vi "Periodic Tasks.vi"(8 "error in":errorcluster) -> ()   [LabVIEW 2019]
doc: "This VI runs in parallel to other tasks. It can contain as many user-defined periodic loops as you need. These can carry out PID or other sorts of timed response."
uses:
  <vilib>/Rock Robotics/WPI/DriverStation/WPI_DriverStationRobotMode2.ctl
  Robot Global Data.vi
  <vilib>/Rock Robotics/WPI/Utilities/WPI_GetSetVariantRefNum.vi
  <vilib>/Rock Robotics/Network Tables/NT Write Boolean.vi
  <vilib>/Rock Robotics/Network Tables/NT Write Number.vi
  <vilib>/Rock Robotics/Network Tables/NT Read Number.vi
  <vilib>/Rock Robotics/WPI/RobotDrive/WPI_RobotDriveArcadeDrive_Standard(NoSaturation).vi
  <vilib>/Rock Robotics/Network Tables/NT Read Boolean.vi
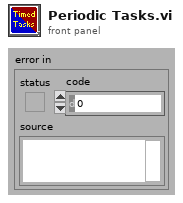
[diagram p1: front panel]
types:
  T1 = typedef "WPI_JoystickDevRef.ctl" = cluster{"Device":T2}
  T2 = typedef "WPI_JoystickDeviceEnum.ctl" = enum16{"USB 0", "USB 1", "USB 2", "USB 3", "USB 4", "USB 5"}
  T3 = typedef "WPI_RobotDriveDevRef.ctl" = cluster{"DevStatus":errorcluster, "Motors[]":T4[], "Square Inputs":bool, "Max Output":dbl}
  T4 = typedef "WPI_MotorControlDeviceRef.ctl" = cluster{"DeviceStatus":errorcluster, "Type":T5, "PWM":cluster{"PWM Channel":T6, "DeadBand":T7}, "CAN":cluster{"Device Number":u8, "SetOutput VI Ref":variant, "GetOutput VI Ref":variant, "Enable VI Ref":variant, "Disable VI Ref":variant, "Data":variant}, "Invert":bool, "DIO PWM":cluster{"PWM \"Enable\" Channel":T6, "DIOChannel":T8, "PWM Rate":dbl}}
  T5 = typedef "WPI_MotorControlType.ctl" = enum16{"PWM", "CAN", "DIO PWM"}
  T6 = typedef "FPGA_DIOPWMChannel.ctl" = enum8{"PWM 0", "PWM 1", "PWM 2", "PWM 3", "PWM 4", "PWM 5", "PWM 6", "PWM 7", "PWM 8", "PWM 9", "PWM MXP 0", "PWM MXP 1", "PWM MXP 2", "PWM MXP 3", "PWM MXP 4", "PWM MXP 5", "PWM MXP 6", "PWM MXP 7", "PWM MXP 8", "PWM MXP 9", "Invalid"}
  T7 = typedef "WPI_PWMDeadband.ctl" = cluster{"Name":string, "maxPositivePwm":i32, "minPositivePwm":i32, "centerPwm":i32, "maxNegativePwm":i32, "minNegativePwm":i32, "angularRange":u16}
  T8 = typedef "FPGA_DIOChannel.ctl" = enum8{"DIO 0", "DIO 1", "DIO 2", "DIO 3", "DIO 4", "DIO 5", "DIO 6", "DIO 7", "DIO 8", "DIO 9", "DIO MXP 0", "DIO MXP 1", "DIO MXP 2", "DIO MXP 3", "DIO MXP 4", "DIO MXP 5", "DIO MXP 6", "DIO MXP 7", "DIO MXP 8", "DIO MXP 9", "DIO MXP 10", "DIO MXP 11", "DIO MXP 12", "DIO MXP 13", "DIO MXP 14", "DIO MXP 15", "SPI Port CS1", "SPI Port CS2", "SPI Port CS3", "SPI Port MISO", "SPI Port MOSI", "Invalid"}
  T9 = cluster{"JoystickDevRef":T1, "RobotDriveDevRef":T3}
  T10 = typedef "WPI_DriverStationRobotMode2.ctl" = enum16{"Autonomous Disabled", "Autonomous Enabled", "Teleop Disabled", "Teleop Enabled", "Disconnected", "Finish", "Test Disabled", "Test Enabled", "Emergency Stopped"}
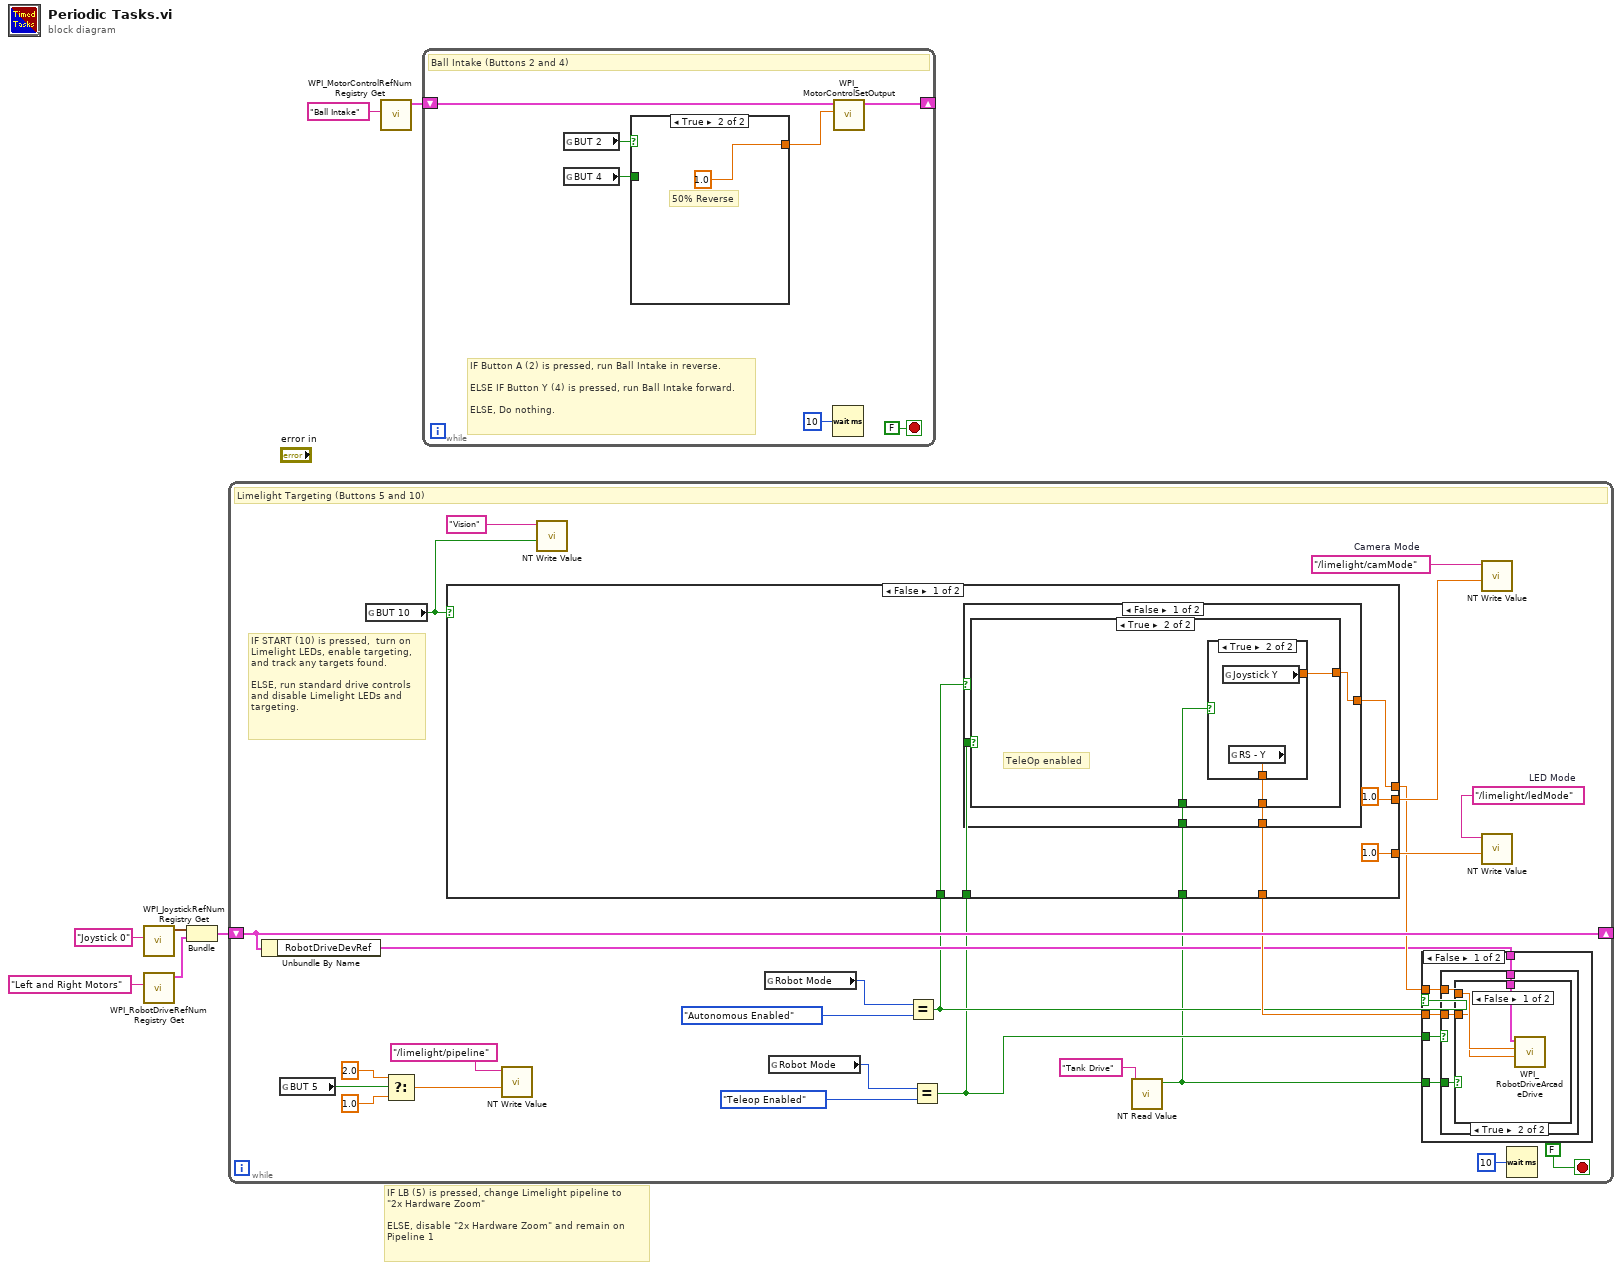
[diagram p0: block diagram]
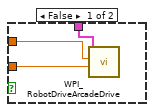
[diagram p2: hidden frame]
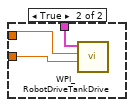
[diagram p3: hidden frame]
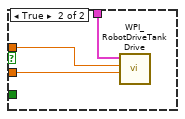
[diagram p4: hidden frame]
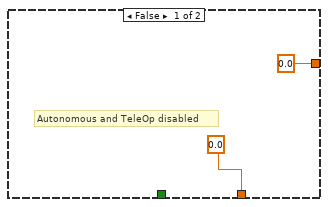
[diagram p5: hidden frame]
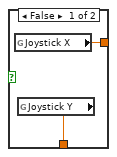
[diagram p6: hidden frame]
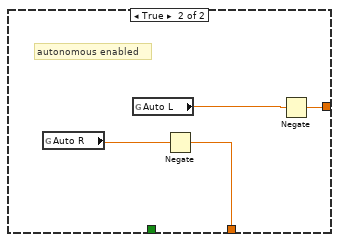
[diagram p7: hidden frame]
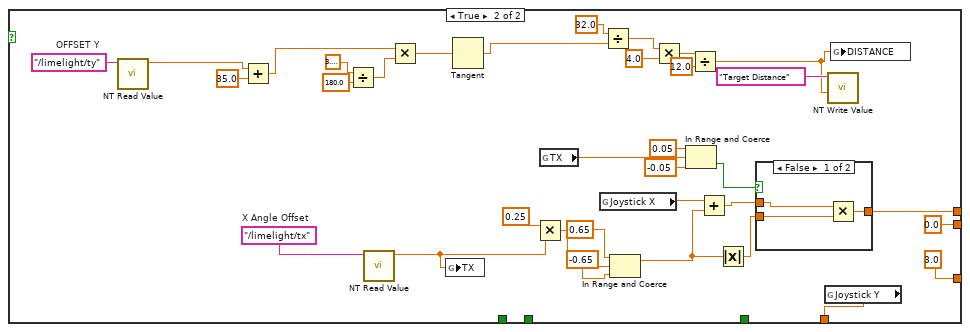
[diagram p8: hidden frame]
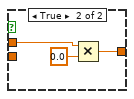
[diagram p9: hidden frame]
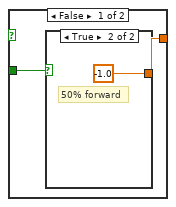
[diagram p10: hidden frame]
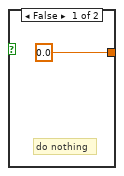
[diagram p11: hidden frame]
diagram:
  # "IF LB (5) is pressed, change Limelight pipeline to \n\"2x Hardware Zoom\"\n\nELSE, disable \"2x Hardware Zoom\" and remain on\nPipeline 1"
  n1 = call <vilib>:"WPI_JoystickRefNum Registry Get.vi"("refnum name"="Joystick 0") -> ("JoystickDevRef"=w3:T1)  [unwired: 1 in, 9 out]
  n2 = call <vilib>:"WPI_RobotDriveRefNum Registry Get.vi"("refnum name"="Left and Right Motors") -> ("RobotDriveDevRef"=w2:T3)  [unwired: 1 in, 9 out]
  n3 = Bundle("JoystickDevRef"=w3, "RobotDriveDevRef"=w2) -> (w1:T9)  [unwired: 1 out]
  n4 = while {
    shift-right: [w31] -> _
    shift-left: w1 -> [w31]
    stop <- FALSE stop-if-true
    w29 = "/limelight/camMode"  # Camera Mode
    w30 = "/limelight/ledMode"  # LED Mode
    # "IF START (10) is pressed,  turn on\nLimelight LEDs, enable targeting,\nand track any targets found.\n\nELSE, run standard drive controls\nand disable Limelight LEDs and \ntargeting."
    # "Limelight Targeting (Buttons 5 and 10)"
    n5 = Unbundle By Name(w31) -> ("RobotDriveDevRef"=w16:T3)
    n6 = global read "Robot Global Data.vi" "BUT 5"() -> (w19:bool)
    n7 = global read "Robot Global Data.vi" "BUT 10"() -> (w25:bool)
    n8 = Select(t=2.0, s=w19, f=1.0) -> (s? t:f=w22:dbl)
    n9 = call-poly <vilib>:"NT Write Value.vi"("Numeric"=w22, "Name"="/limelight/pipeline") -> ()  [unwired: 9 in, 1 out]
    n10 = call-poly <vilib>:"NT Write Value.vi"("Boolean"=w25, "Name"="Vision") -> ()  [unwired: 9 in, 1 out]
    n11 = global read "Robot Global Data.vi" "Robot Mode"() -> (w15:T10)
    n12 = global read "Robot Global Data.vi" "Robot Mode"() -> (w11:T10)
    n13 = Equal?(x=w15, y=WPI_DriverStationRobotMode2."Autonomous Enabled") -> (x = y?=w13:bool)
    n14 = Equal?(x=w11, y=WPI_DriverStationRobotMode2."Teleop Enabled") -> (x = y?=w10:bool)
    n15 = call-poly <vilib>:"NT Read Value.vi"("Name"="Tank Drive") -> ("Boolean"=w8:bool)  [unwired: 9 in, 1 out]
    n16 = case shown="False" w25 {
      tunnel: [1.0 ("Numeric") 0.0 ("Numeric")] -> w28
      tunnel: [1.0 ("Numeric") 3.0 ("Numeric")] -> w27
      tunnel: [w57 w104] -> w17
      tunnel: [w58 w103] -> w18
      tunnel: w13 -> [w56 _]
      tunnel: w10 -> [w55 _]
      tunnel: w8 -> [w54 _]
      frame False {
        n17 = case shown="False" w56 {
          tunnel: [w63 w75] -> w58
          tunnel: [w64 w77] -> w57
          tunnel: w55 -> [w62 _]
          tunnel: w54 -> [w61 _]
          frame False {
            n18 = case shown="True" w62 {
              tunnel: [0.0 ("Joystick X") w69] -> w64
              tunnel: [0.0 ("Joystick Y") w68] -> w63
              tunnel: w61 -> [_ w67]
              frame False {
                # "Autonomous and TeleOp disabled"
              }
              frame True {
                # "TeleOp enabled"
                n19 = case shown="True" w67 {
                  tunnel: [w71 w73] -> w69
                  tunnel: [w70 w72] -> w68
                  frame False {
                    n20 = global read "Robot Global Data.vi" "Joystick X"() -> (w71:dbl)
                    n21 = global read "Robot Global Data.vi" "Joystick Y"() -> (w70:dbl)
                  }
                  frame True {
                    n22 = global read "Robot Global Data.vi" "Joystick Y"() -> (w73:dbl)
                    n23 = global read "Robot Global Data.vi" "RS - Y"() -> (w72:dbl)
                  }
                }
              }
            }
          }
          frame True {
            # "autonomous enabled"
            n24 = global read "Robot Global Data.vi" "Auto R"() -> (w74:dbl)
            n25 = global read "Robot Global Data.vi" "Auto L"() -> (w76:dbl)
            n26 = Negate(x=w74) -> (-x=w75:dbl)
            n27 = Negate(x=w76) -> (-x=w77:dbl)
          }
        }
      }
      frame True {
        w87 = "/limelight/ty"  # OFFSET Y
        w105 = "/limelight/tx"  # X Angle Offset
        n28 = call-poly <vilib>:"NT Read Value.vi"("Name"=w87) -> ("Numeric"=w85:dbl)  [unwired: 9 in, 1 out]
        n29 = Add(x=w85, y=35.0) -> (x+y=w83:dbl)
        n30 = Divide(x=3.141592653589793, y=180.0) -> (x/y=w93:dbl)
        n31 = call-poly <vilib>:"NT Read Value.vi"("Name"=w105) -> ("Numeric"=w109:dbl)  [unwired: 9 in, 1 out]
        n32 = Multiply(x=w83, y=w93) -> (x*y=w92:dbl)
        n33 = global write "Robot Global Data.vi" "TX"(w109) -> ()
        n34 = Tangent(1:w92) -> (0:w91:dbl)
        n35 = Multiply(x=0.25 ("y"), y=w109) -> (x*y=w106:dbl)
        n36 = global read "Robot Global Data.vi" "TX"() -> (w99:dbl)
        n37 = global read "Robot Global Data.vi" "Joystick X"() -> (w97:dbl)
        n38 = Divide(x=32.0, y=w91) -> (x/y=w82:dbl)
        n39 = In Range and Coerce(upper limit=0.65, x=w106, lower limit=-0.65) -> (coerced(x)=w94:dbl)  [unwired: 1 out]
        n40 = Multiply(x=w82, y=4.0) -> (x*y=w80:dbl)
        n41 = In Range and Coerce(upper limit=0.05, x=w99, lower limit=-0.05) -> (In Range?=w102:bool)  [unwired: 1 out]
        n42 = Divide(x=w80, y=12.0) -> (x/y=w78:dbl)
        n43 = Add(x=w97, y=w94) -> (x+y=w96:dbl)
        n44 = Absolute Value(x=w94) -> (abs(x)=w95:dbl)
        n45 = case shown="False" w102 {
          tunnel: [w114 w116] -> w104
          tunnel: w96 -> [w113 w115]
          tunnel: w95 -> [w112 _]
          frame False {
            n46 = Multiply(x=w113, y=w112) -> (x*y=w114:dbl)
          }
          frame True {
            n47 = Multiply(x=w115, y=0.0) -> (x*y=w116:dbl)
          }
        }
        n48 = global read "Robot Global Data.vi" "Joystick Y"() -> (w103:dbl)
        n49 = call-poly <vilib>:"NT Write Value.vi"("Numeric"=w78, "Name"="Target Distance") -> ()  [unwired: 9 in, 1 out]
        n50 = global write "Robot Global Data.vi" "DISTANCE"(w78) -> ()
      }
    }
    n51 = case shown="False" w13 {
      tunnel: w18 -> [w37 w51]
      tunnel: w17 -> [w36 w52]
      tunnel: w16 -> [w35 w53]
      tunnel: w10 -> [w34 _]
      tunnel: w8 -> [w33 _]
      frame False {
        n52 = case shown="True" w34 {
          tunnel: w37 -> [w39 w44]
          tunnel: w36 -> [w40 w43]
          tunnel: w35 -> [w38 w42]
          tunnel: w33 -> [_ w41]
          frame False {
            n53 = call-poly <vilib>:"WPI_RobotDriveArcadeDrive.vi"("Y axis value"=w39, "X axis value"=w40, "RobotDriveDevRef"=w38) -> ()  [unwired: 6 in, 3 out]
          }
          frame True {
            n54 = case shown="False" w41 {
              tunnel: w44 -> [w45 w50]
              tunnel: w43 -> [w46 w49]
              tunnel: w42 -> [w47 w48]
              frame False {
                n55 = call-poly <vilib>:"WPI_RobotDriveArcadeDrive.vi"("Y axis value"=w45, "X axis value"=w46, "RobotDriveDevRef"=w47) -> ()  [unwired: 6 in, 3 out]
              }
              frame True {
                n56 = call <vilib>:"WPI_RobotDriveTankDrive.vi"("Right axis value"=w50, "Left axis value"=w49, "RobotDriveDevRef"=w48) -> ()  [unwired: 6 in, 3 out]
              }
            }
          }
        }
      }
      frame True {
        n57 = call <vilib>:"WPI_RobotDriveTankDrive.vi"("Right axis value"=w51, "Left axis value"=w52, "RobotDriveDevRef"=w53) -> ()  [unwired: 6 in, 3 out]
      }
    }
    n58 = call-poly <vilib>:"NT Write Value.vi"("Numeric"=w28, "Name"=w29) -> ()  [unwired: 9 in, 1 out]
    n59 = call-poly <vilib>:"NT Write Value.vi"("Numeric"=w27, "Name"=w30) -> ()  [unwired: 9 in, 1 out]
    n60 = Wait (ms)(milliseconds to wait=u32 10) -> ()  [unwired: 1 out]
  }
  n61 = call <vilib>:"WPI_MotorControlRefNum Registry Get.vi"("refnum name"="Ball Intake") -> ("MotorControlDevRef"=w7:T4)  [unwired: 9 in, 1 out]
  n62 = while {
    shift-right: [w121] -> _
    shift-left: w7 -> [w120]
    stop <- FALSE stop-if-true
    # "IF Button A (2) is pressed, run Ball Intake in reverse. \n\nELSE IF Button Y (4) is pressed, run Ball Intake forward.\n\nELSE, Do nothing."
    # "Ball Intake (Buttons 2 and 4)"
    n63 = global read "Robot Global Data.vi" "BUT 2"() -> (w123:bool)
    n64 = global read "Robot Global Data.vi" "BUT 4"() -> (w124:bool)
    n65 = case shown="True" w123 {
      tunnel: [w126 1.0 ("Output")] -> w122
      tunnel: w124 -> [w125 _]
      frame False {
        n66 = case shown="True" w125 {
          tunnel: [0.0 ("Output") -1.0 ("Output")] -> w126
          frame False {
            # "do nothing"
          }
          frame True {
            # "50% forward"
          }
        }
      }
      frame True {
        # "50% Reverse"
      }
    }
    n67 = Wait (ms)(milliseconds to wait=u32 10) -> ()  [unwired: 1 out]
    n68 = call <vilib>:"WPI_MotorControlSetOutput.vi"("Output"=w122, "MotorControlDevRef"=w120) -> ("MotorControlDevRef"=w121:T4)  [unwired: 7 in, 2 out]
  }
